vi "eFGV - Start Acquisition.vi"(6 "FGV State":T1, 8 "Error In":errorcluster, 11 "Start Test":bool) -> (0 "Error Out":errorcluster, 2 "Event Start Acquire":refnum<user-event>, 3 "Start Out":bool)   [LabVIEW 2020]
uses:
  Control/State - eFGV.ctl
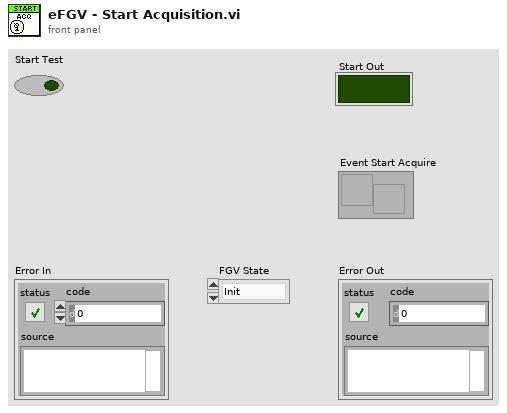
[diagram p1: front panel]
types:
  T1 = typedef "State - eFGV.ctl" = enum16{"Init", "Read", "Write", "Exit"}
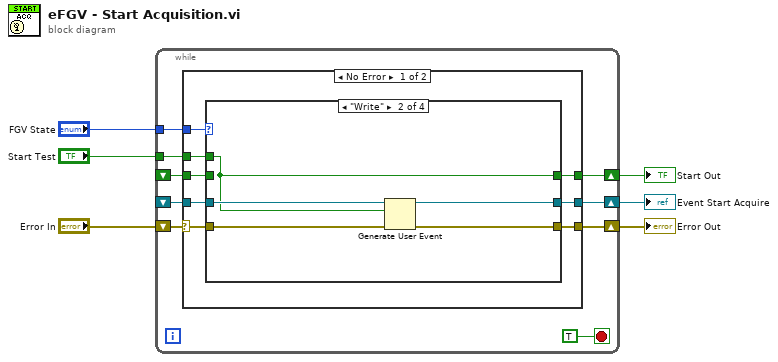
[diagram p0: block diagram]
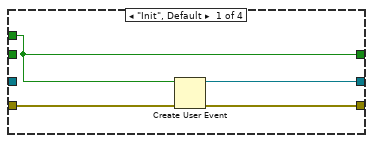
[diagram p2: hidden frame]
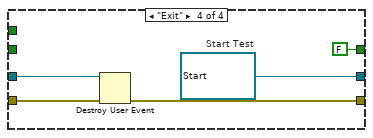
[diagram p4: hidden frame]
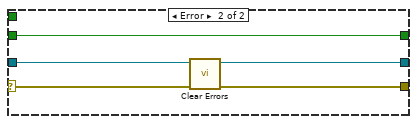
[diagram p5: hidden frame]
diagram:
  n1 = while {
    shift-right: [w14] -> w5
    shift-left: "Error In" -> [w15]
    tunnel: "FGV State" -> [w13]
    tunnel: "Start Test" -> [w11]
    shift-right: [w10] -> w1
    shift-left: _ -> [w8]
    shift-right: [w9] -> w2
    shift-left: _ -> [w7]
    stop <- TRUE stop-if-true
    n2 = case shown="No Error" w15 {
      selector: w15 -> [w23 w44]
      tunnel: w13 -> [w21 _]
      tunnel: w11 -> [w20 _]
      tunnel: [w22 w43] -> w14
      tunnel: [w19 w41] -> w10
      tunnel: [w18 w42] -> w9
      tunnel: w8 -> [w17 w41]
      tunnel: w7 -> [w16 w42]
      frame No Error {
        n3 = case shown="\"Write\"" w21 {
          tunnel: w20 -> [w24 w28 _ _]
          tunnel: w23 -> [w27 w32 w35 w40]
          tunnel: [w26 w31 w35 w39] -> w22
          tunnel: [w25 w30 w34 w37] -> w19
          tunnel: [w24 w28 w33 FALSE ("Start")] -> w18
          tunnel: w17 -> [_ w29 w34 w38]
          tunnel: w16 -> [_ _ w33 _]
          frame "Init", Default {
            n4 = Create User Event(user event datatype=w24, error in=w27) -> (user event=w25:refnum<user-event>, error out=w26:errorcluster)
          }
          frame "Write" {
            n5 = Generate User Event(user event=w29, event data cluster=w28, error in=w32) -> (user event out=w30:refnum<user-event>, error out=w31:errorcluster)  [unwired: 1 in]
          }
          frame "Read" {
          }
          frame "Exit" {
            w37 = refnum<user-event> refnum  # Start Test
            n6 = Destroy User Event(user event=w38, error in=w40) -> (error out=w39:errorcluster)
          }
        }
      }
      frame Error {
        n7 = call <vilib>:"Clear Errors.vi"("error in (no error)"=w44) -> ("error out"=w43:errorcluster)  [unwired: 5 in, 1 out]
      }
    }
  }
  "Start Out" <- w2
  "Error Out" <- w5
  "Event Start Acquire" <- w1
